vi "State Logic.vi"(0 "TLB' data in":refnum<class "{TMPL} TLB`.lvclass">, 1 "process state logic enable":bool, 5 "trigger queue in":refnum<queue>, 7 "action queue in":refnum<queue>, 11 "error in":errorcluster) -> (4 "TLB' data out":refnum<class "{TMPL} TLB`.lvclass">, 15 "error out":errorcluster)   [LabVIEW 2018, in "TLB` Template.lvlib" / "{TMPL} TLB`.lvclass"]
doc: "Control process for TLB' template.\n\n<B>Input Parameters</B>\n\n<B>TLB' data in</B> is the templates' private data.\n\n<B>process state logic enable</B> enable state logic change.\n\n<B>trigger queue in</B> is a reference to a queue. Use the Create Trigger Queue function to obtain a queue reference. \n\n<B>action queue in</B> is a reference to a queue. Use the Create Action Queue function to obtain a queue reference. \n\n<B>timeout (ms)</B> queue timeout.\n\n<B>error in</B> describes error conditions that occur before this node runs. This input provides standard error in functionality.\n\n<B>Output Parameters</B>\n\n<B>TLB' data out</B> is the templates' private data.\n\n<B>error out</B> contains error information. This output provides standard error out functionality."
uses:
  {TMPL} TLB`.lvclass
  Application Components/Trigger API/System Trigger Element.ctl
  Application Components/Trigger API/System Trigger.ctl
  Core Components/Actions/System Action Element.ctl
  {TMPL} TLB`.lvclass/{TMPL} TLB`.ctl
  State.ctl
  Core Components/Error Handler/TLB` Error Handler.lvclass/TLB` Error Handler.ctl
  Core Components/Error Handler/accessors/Get Action Causing Error.vi
  Core Components/Error Handler/accessors/Get Originating State.vi
  Core Components/Error Handler/accessors/Get Destination State.vi
  Core Components/Error Handler/accessors/Get Executed System Actions.vi
  Core Components/Error Handler/accessors/Get Remaing System Actions.vi
  Core Components/Error Handler/Core/actions/support/Error FLUSH-LOG-DIALOG.vi
  Core Components/Error Handler/Core/actions/support/Error FLUSH-DIALOG.vi
  Application Components/Trigger API/{TMPL} Trigger API.lvlib
  Core Components/Error Handler/TLB` Error Handler.lvclass
  Core Components/Actions/Actions.lvlib
  TLB` Template.lvlib
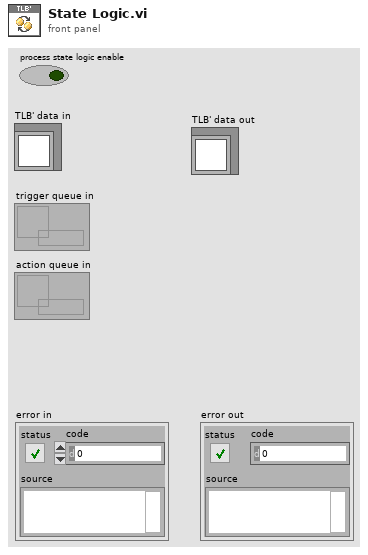
[diagram p1: front panel]
types:
  T1 = typedef "TLB` Template.lvlib/{TMPL} TLB`.lvclass/State.ctl" = enum16{"<Startup>", "Idle", "Connected", "Monitoring", "Sweeping", "<Shutdown>", "<Error>"}
  T2 = typedef "TLB` Template.lvlib/{TMPL} Trigger API.lvlib/System Trigger.ctl" = enum16{"<None>", "Connect", "Start Acquisition", "Stop Acquisition", "Disconnect", "Load Configuration", "Save Configuration", "<Return to Safe State Actions>", "<Cache User Parameters>", "<Close Application>", "<Error>"}
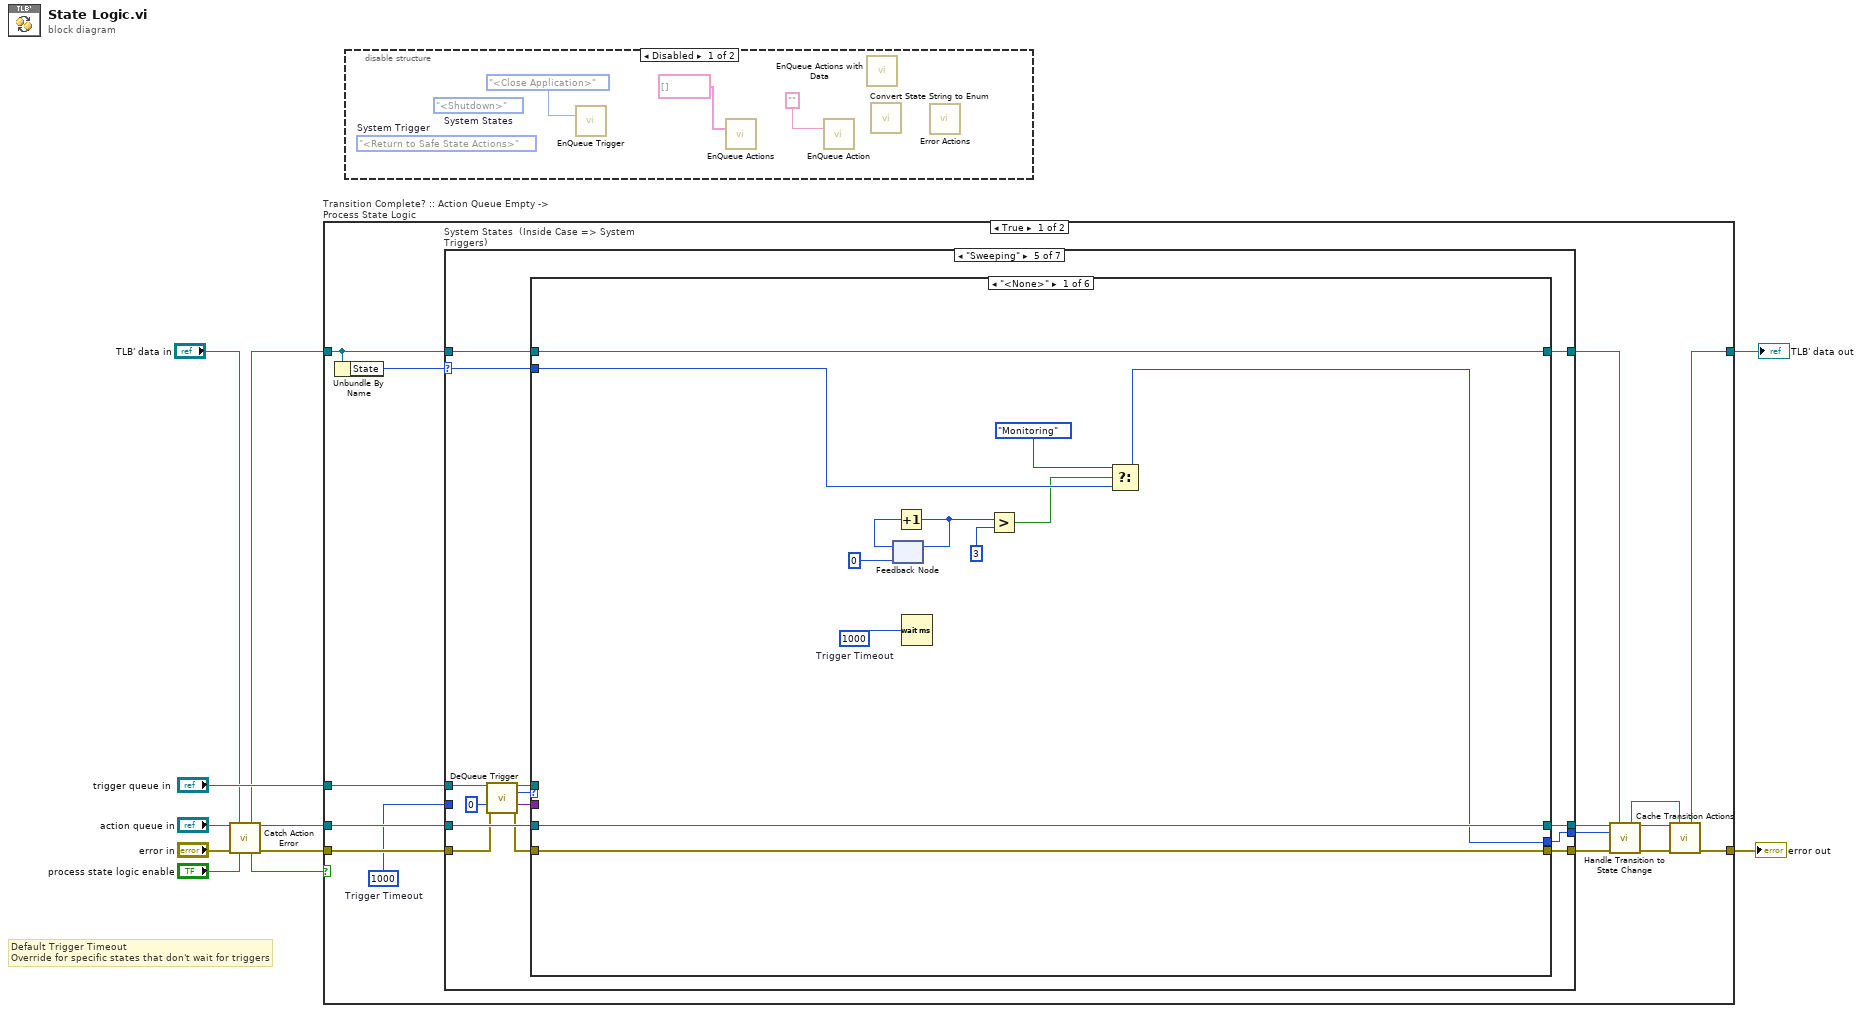
[diagram p0: block diagram]
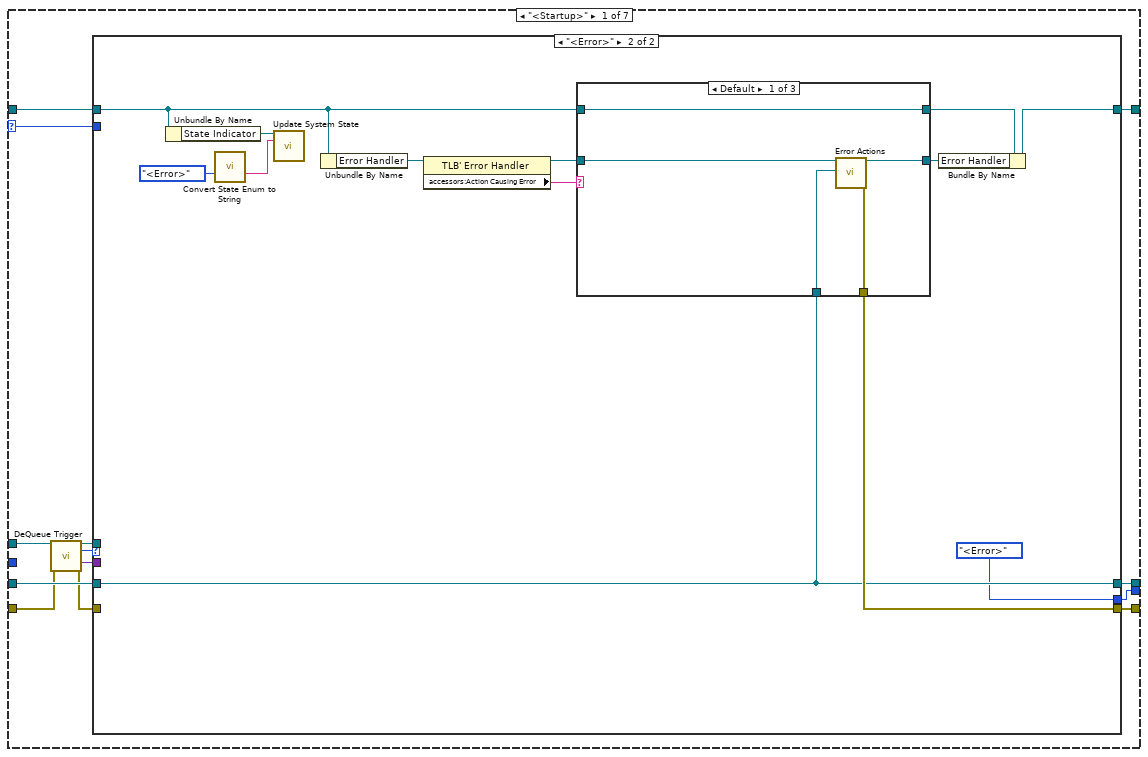
[diagram p3: hidden frame]
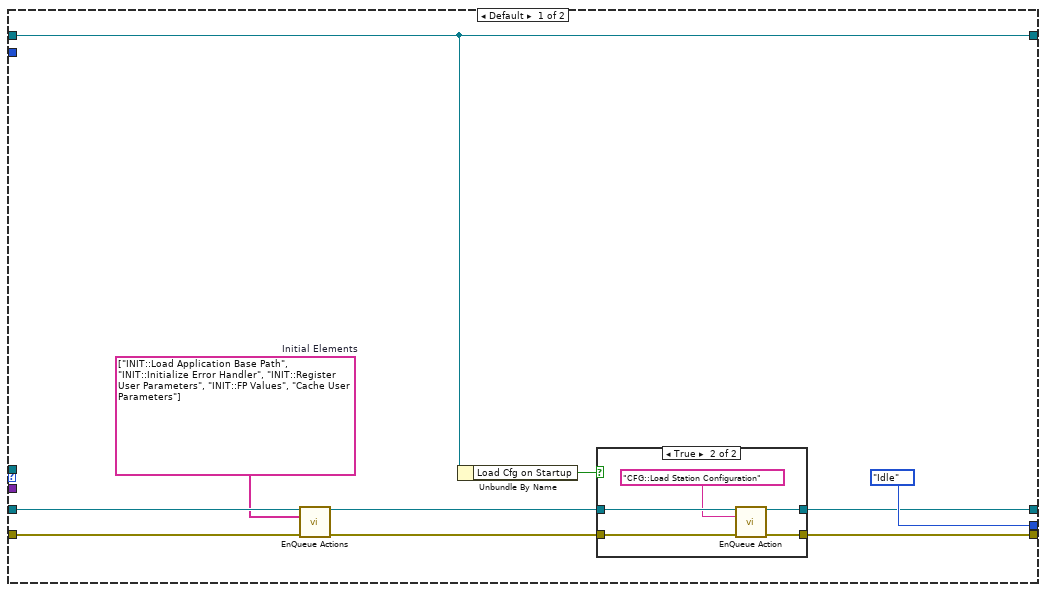
[diagram p4: hidden frame]
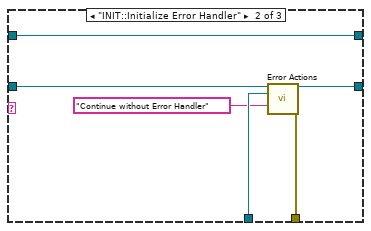
[diagram p6: hidden frame]
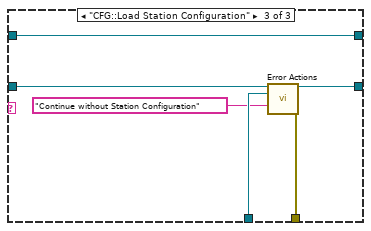
[diagram p7: hidden frame]
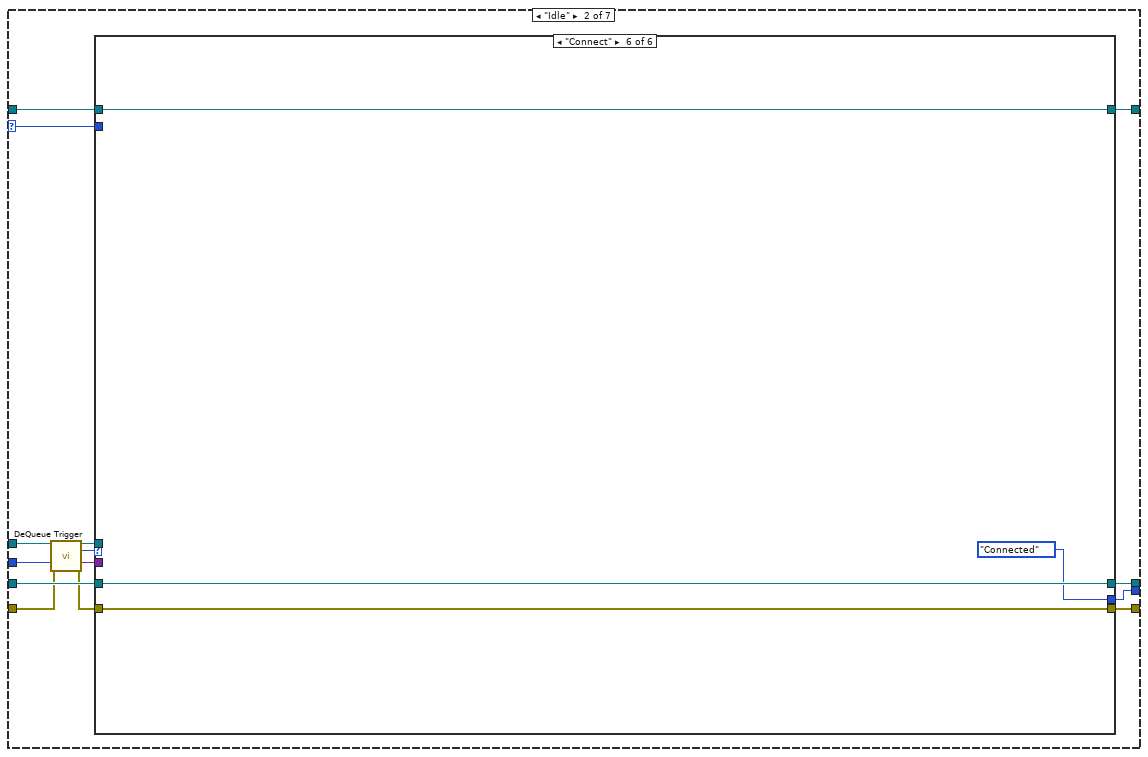
[diagram p8: hidden frame]
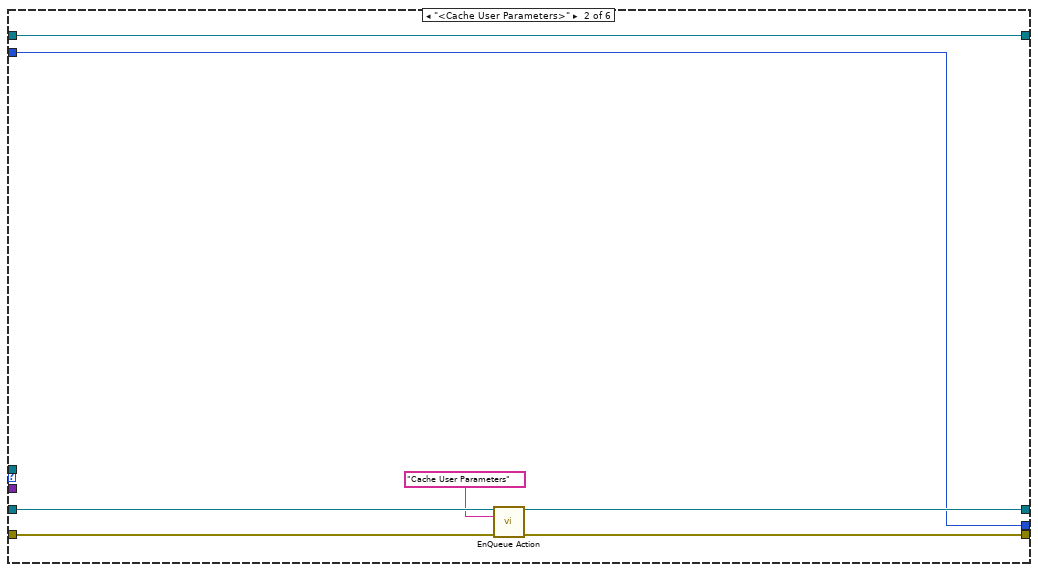
[diagram p10: hidden frame]
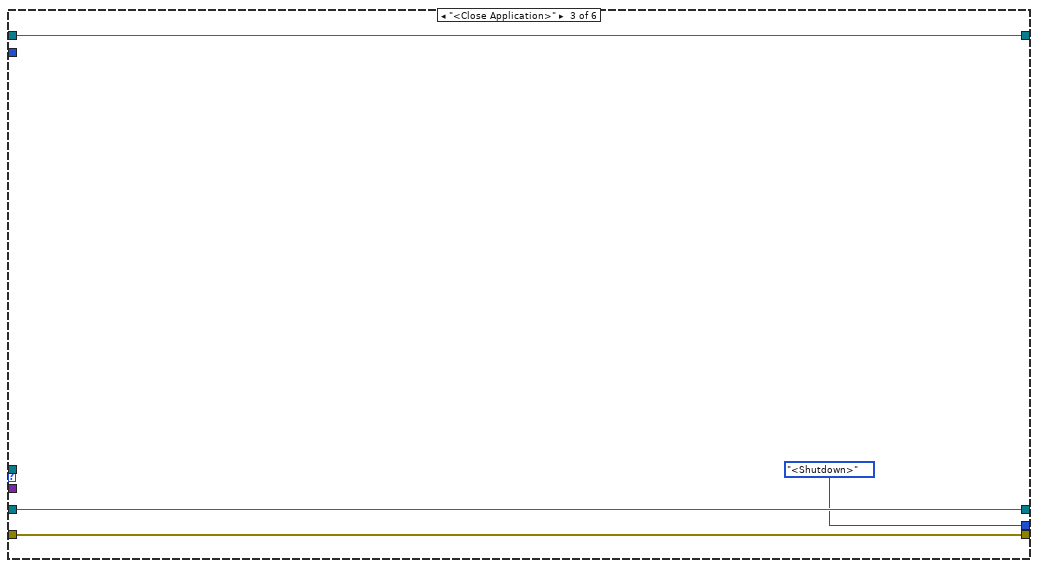
[diagram p11: hidden frame]
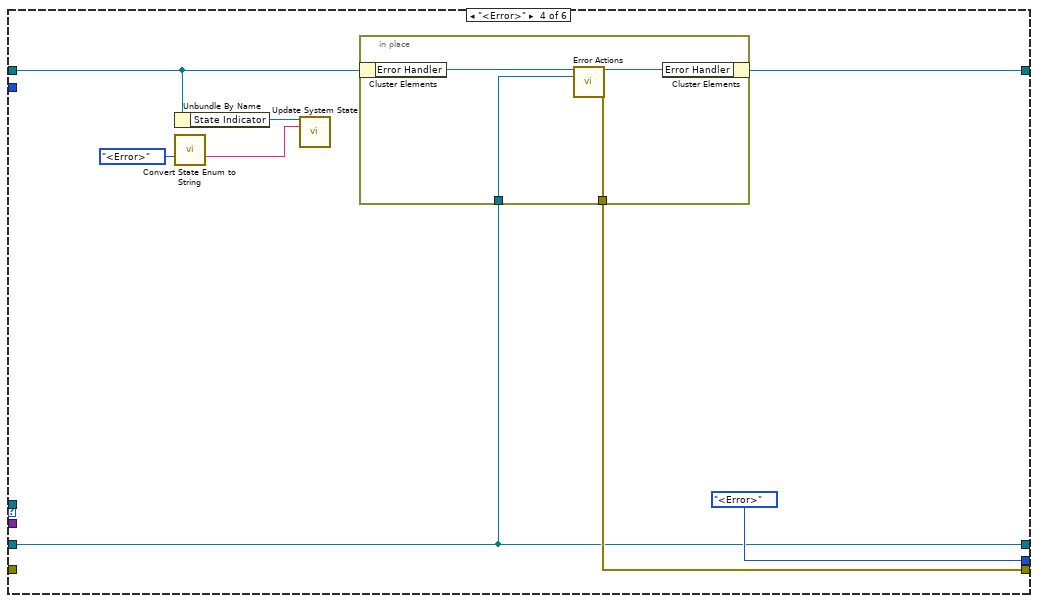
[diagram p12: hidden frame]
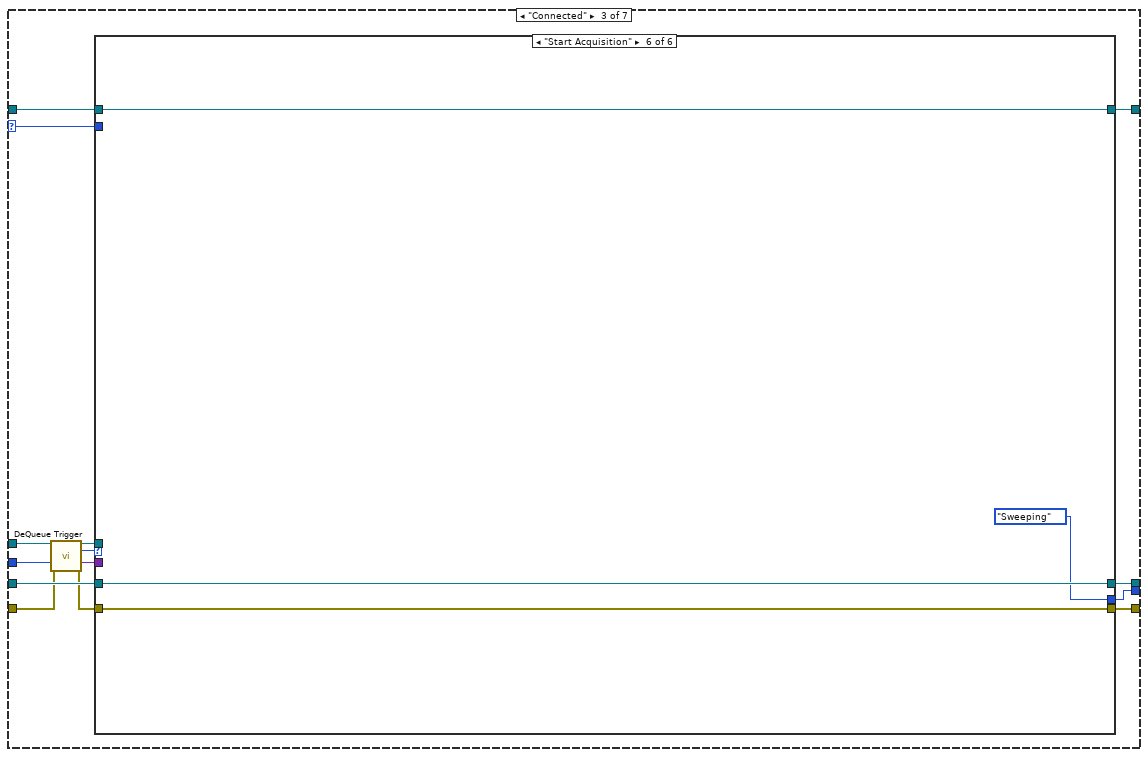
[diagram p14: hidden frame]
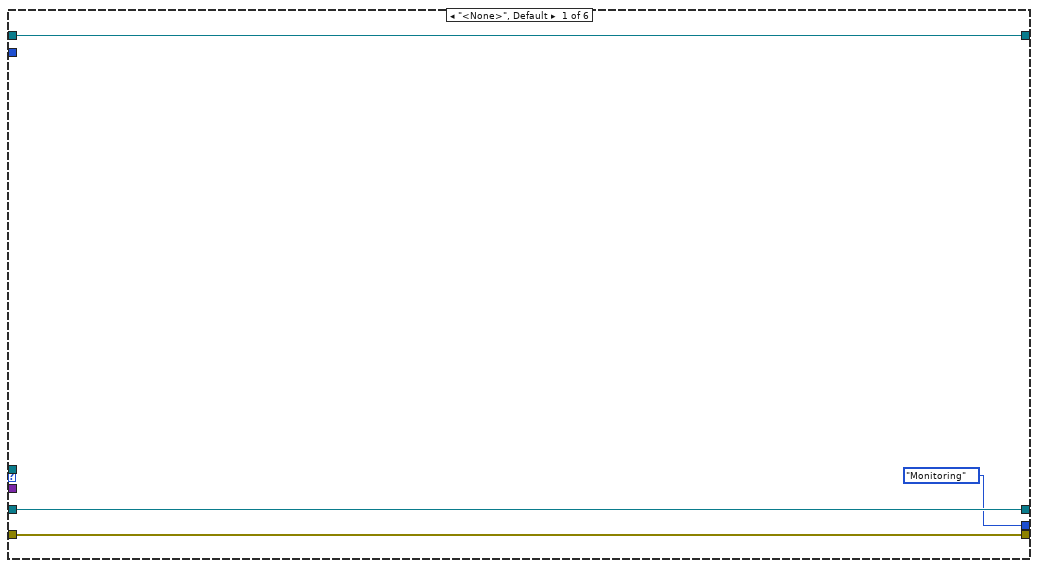
[diagram p15: hidden frame]
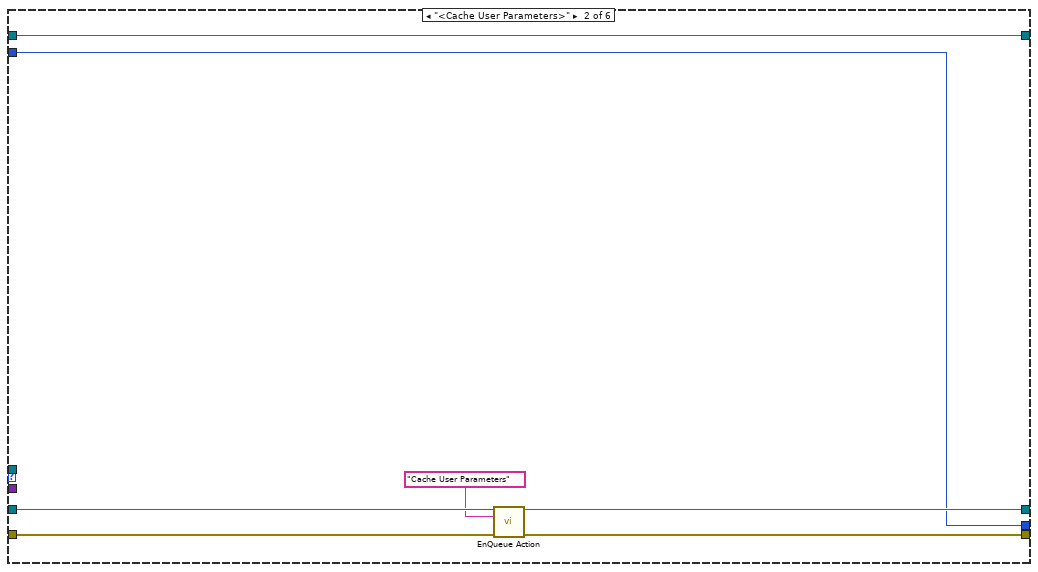
[diagram p16: hidden frame]
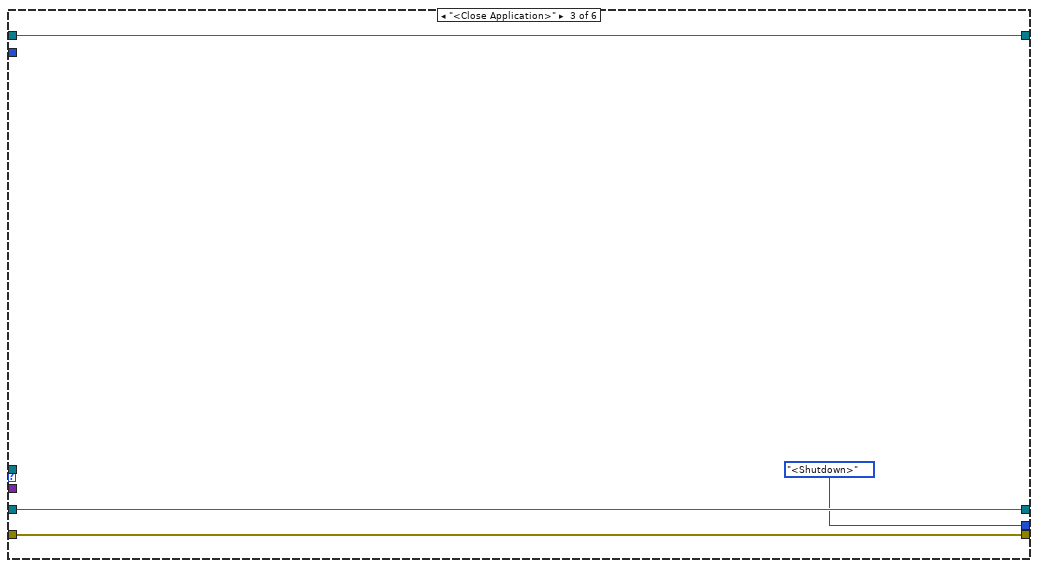
[diagram p17: hidden frame]
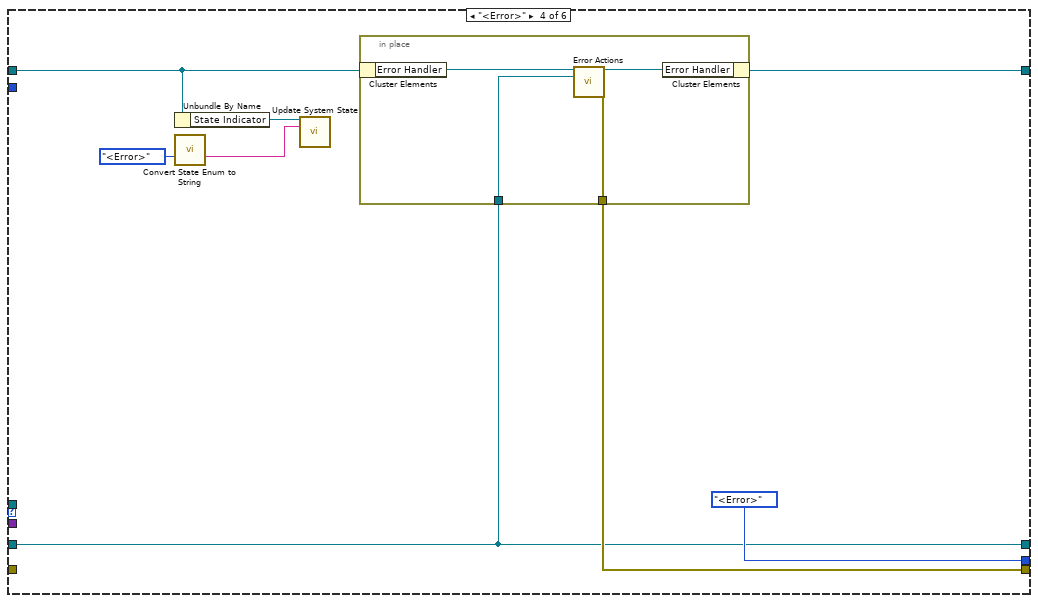
[diagram p18: hidden frame]
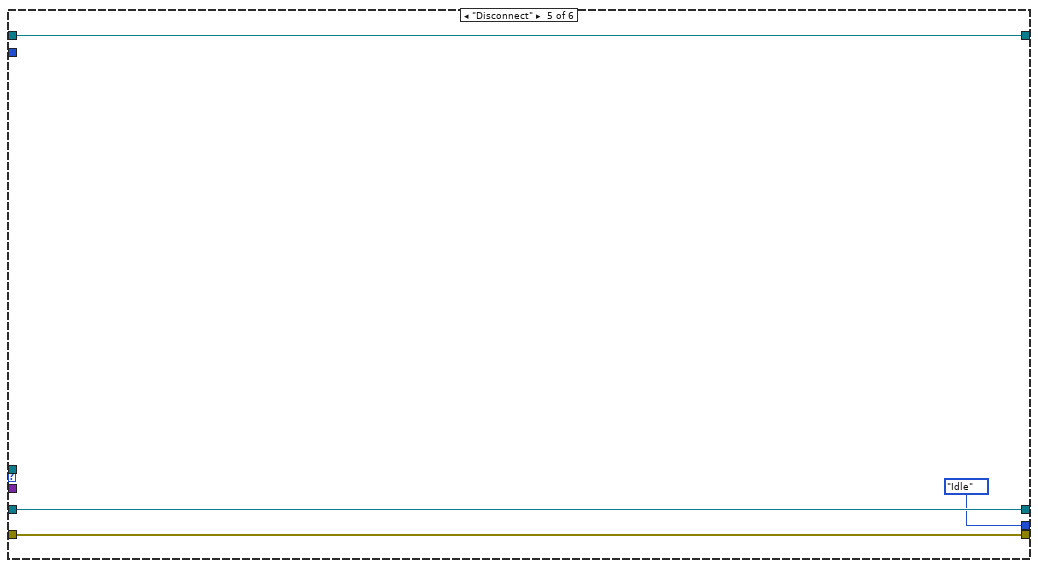
[diagram p19: hidden frame]
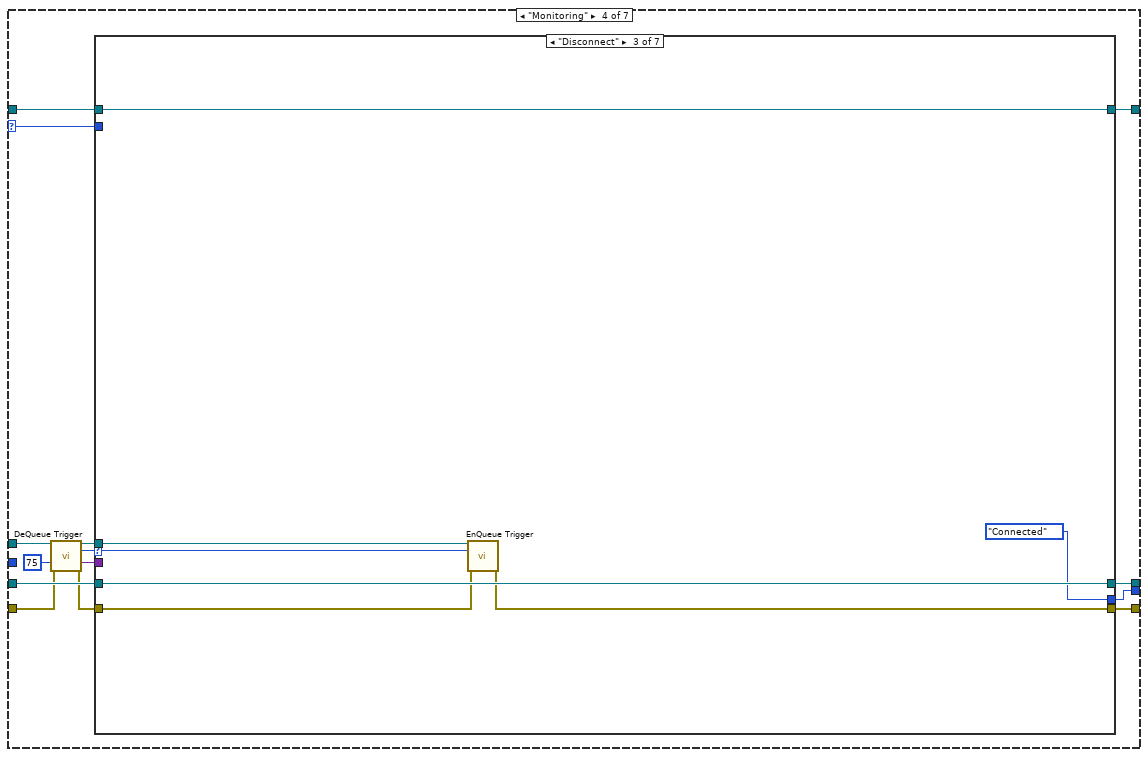
[diagram p20: hidden frame]
diagram:
  # "Default Trigger Timeout\nOverride for specific states that don't wait for triggers"
  n1 = call "Catch Action Error.vi"("action queue in"="action queue in", "TLB' Template in"="TLB' data in", "error in (no error)"="error in", "process state logic enable in"="process state logic enable") -> ("TLB' Template out"=w6:refnum<class "{TMPL} TLB`.lvclass">, "action queue in"=w2:refnum<queue>, "process state logic enable out"=w4:bool, "error out"=w7:errorcluster)  [unwired: 8 in]
  n2 = case "Transition Complete? :: Action Queue Empty -> Process State Logic" shown="True" w4 {
    tunnel: [w17 w404] -> w10
    tunnel: w6 -> [w22 w404]
    tunnel: w7 -> [w26 w405]
    tunnel: w2 -> [w25 _]
    tunnel: [w20 w405] -> w11
    tunnel: "trigger queue in" -> [w24 _]
    frame True {
      w18 = 1000  # Trigger Timeout
      n3 = Unbundle By Name(w22) -> ("State"=w19:T1)
      n4 = case "System States  (Inside Case => System Triggers)" shown="\"Sweeping\"" w19 {
        selector: w19 -> [w27 w89 w138 w187 w243 w305 _]
        tunnel: [w33 w94 w143 w192 w248 w303 w402] -> w15
        tunnel: w22 -> [w34 w95 w144 w193 w249 w304 w402]
        tunnel: w26 -> [w32 w93 w142 w191 w247 w302 w401]
        tunnel: w25 -> [w38 w99 w148 w197 w253 w306 w400]
        tunnel: [w37 w98 w147 w196 w252 w309 w398] -> w23
        tunnel: w24 -> [w39 w100 w149 w198 w254 w310 _]
        tunnel: [w36 w97 w146 w195 w251 w308 w399] -> w16
        tunnel: [w35 w96 w145 w194 w250 w307 State."<Shutdown>" ("State")] -> w12
        tunnel: w18 -> [_ w88 w137 _ _ _ _]
        frame "<Startup>" {
          n5 = call "DeQueue Trigger.vi"("trigger queue in"=w39, "error in"=w32) -> ("trigger queue out"=w28:refnum<queue>, "system trigger"=w30:T2, "trigger data"=w29:variant, "error out"=w31:errorcluster)  [unwired: 10 in]
          n6 = case shown="\"<Error>\"" w30 {
            tunnel: w31 -> [w46 _]
            tunnel: w38 -> [w48 w67]
            tunnel: [w43 w68] -> w37
            tunnel: [w41 w67] -> w36
            tunnel: w29 -> [_ _]
            tunnel: [State."Idle" ("State") State."<Error>" ("State")] -> w35
            tunnel: w34 -> [w44 w58]
            tunnel: [w44 w69] -> w33
            tunnel: w28 -> [_ _]
            tunnel: w27 -> [_ _]
            frame Default {
              w47 = string[] ["INIT::Load Application Base Path", "INIT::Initialize Error Handler", "INIT::Register User Parameters", "INIT::FP Values", "Cache User Parameters"]  # Initial Elements
              n7 = call "EnQueue Actions.vi"("action queue in"=w48, "actions"=w47, "error in"=w46) -> ("action queue out"=w42:refnum<queue>, "error out"=w45:errorcluster)  [unwired: 11 in]
              n8 = Unbundle By Name(w44) -> ("Load Cfg on Startup"=w40:bool)
              n9 = case shown="True" w40 {
                tunnel: w45 -> [w50 w56]
                tunnel: [w50 w55] -> w43
                tunnel: w42 -> [w51 w54]
                tunnel: [w51 w53] -> w41
                frame False {
                }
                frame True {
                  n10 = call "EnQueue Action.vi"("action queue in"=w54, "action"="CFG::Load Station Configuration", "error in"=w56) -> ("action queue out"=w53:refnum<queue>, "error out"=w55:errorcluster)  [unwired: 11 in]
                }
              }
            }
            frame "<Error>" {
              n11 = Unbundle By Name(w58) -> ("State Indicator"=w62:refnum<user-event>)
              n12 = call "Convert State Enum to String.vi"("state in"=State."<Error>") -> ("state out"=w61:string)  [unwired: 13 in, 1 out]
              n13 = call "Update System State.vi"("State Indicator"=w62, "system state message"=w61) -> ()  [unwired: 13 in, 1 out]
              n14 = Unbundle By Name(w58) -> ("Error Handler"=w64:refnum<class "TLB` Error Handler.lvclass">)
              n15 = property class="TLB' Error Handler"(reference=w64) -> (reference out=w63:refnum<class "TLB` Error Handler.lvclass">, "accessors:Action Causing Error"=w60:string)  [unwired: 1 in, 1 out]
              n16 = case shown="Default" w60 {
                tunnel: [w72 w80 w86] -> w68
                tunnel: w67 -> [w71 w79 w85]
                tunnel: [w73 w78 w84] -> w65
                tunnel: w63 -> [w74 w77 w83]
                tunnel: w58 -> [w70 w75 w81]
                tunnel: [w70 w75 w81] -> w57
                frame Default {
                  n17 = call-poly "Error Actions.vi"("Error Handler in"=w74, "action queue in"=w71) -> ("Error Handler out"=w73:refnum<class "TLB` Error Handler.lvclass">, "error out"=w72:errorcluster)  [unwired: 12 in]
                }
                frame "INIT::Initialize Error Handler" {
                  n18 = call-poly "Error Actions.vi"("Error Handler in"=w77, "action queue in"=w79, "error button text (Return to Safe State)"="Continue without Error Handler") -> ("Error Handler out"=w78:refnum<class "TLB` Error Handler.lvclass">, "error out"=w80:errorcluster)  [unwired: 11 in]
                }
                frame "CFG::Load Station Configuration" {
                  n19 = call-poly "Error Actions.vi"("Error Handler in"=w83, "action queue in"=w85, "error button text (Return to Safe State)"="Continue without Station Configuration") -> ("Error Handler out"=w84:refnum<class "TLB` Error Handler.lvclass">, "error out"=w86:errorcluster)  [unwired: 11 in]
                }
              }
              n20 = Bundle By Name(cluster=w57, "Error Handler"=w65) -> (w69:refnum<class "{TMPL} TLB`.lvclass">)
            }
          }
        }
        frame "Idle" {
          n21 = call "DeQueue Trigger.vi"("trigger queue in"=w100, "timeout, ms (0)"=w88, "error in"=w93) -> ("trigger queue out"=w87:refnum<queue>, "system trigger"=w91:T2, "trigger data"=w90:variant, "error out"=w92:errorcluster)  [unwired: 9 in]
          n22 = case shown="\"Connect\"" w91 {
            tunnel: w92 -> [w103 w111 w114 _ w130 w135]
            tunnel: w99 -> [w104 w108 w115 w119 w131 w134]
            tunnel: [w103 w109 w114 w121 w130 w135] -> w98
            tunnel: [w104 w107 w115 w119 w131 w134] -> w97
            tunnel: w90 -> [_ _ _ _ _ _]
            tunnel: w95 -> [w102 w110 w113 w118 w129 w133]
            tunnel: [w101 w105 State."<Shutdown>" ("State") State."<Error>" ("State") w128 State."Connected" ("State")] -> w96
            tunnel: [w102 w110 w113 w120 w129 w133] -> w94
            tunnel: w89 -> [w101 w105 _ _ w128 _]
            tunnel: w87 -> [_ _ _ _ _ _]
            frame "<None>" {
            }
            frame "<Cache User Parameters>" {
              n23 = call "EnQueue Action.vi"("action queue in"=w108, "action"="Cache User Parameters", "error in"=w111) -> ("action queue out"=w107:refnum<queue>, "error out"=w109:errorcluster)  [unwired: 11 in]
            }
            frame "<Close Application>" {
            }
            frame "<Error>" {
              n24 = Unbundle By Name(w118) -> ("State Indicator"=w122:refnum<user-event>)
              n25 = call "Convert State Enum to String.vi"("state in"=State."<Error>") -> ("state out"=w116:string)  [unwired: 13 in, 1 out]
              n26 = call "Update System State.vi"("State Indicator"=w122, "system state message"=w116) -> ()  [unwired: 13 in, 1 out]
              n27 = in-place {
                in-place-border: [w125] -> w121
                in-place-border: w119 -> [w124]
                n28 = in-place-cluster #1(w118) -> ("Error Handler"=w127:refnum<class "TLB` Error Handler.lvclass">)
                n29 = call-poly "Error Actions.vi"("Error Handler in"=w127, "action queue in"=w124) -> ("Error Handler out"=w126:refnum<class "TLB` Error Handler.lvclass">, "error out"=w125:errorcluster)  [unwired: 12 in]
                n30 = in-place-cluster #1("Error Handler"=w126) -> (w120:refnum<class "{TMPL} TLB`.lvclass">)
              }
            }
            frame Default {
            }
            frame "Connect" {
            }
          }
        }
        frame "Connected" {
          n31 = call "DeQueue Trigger.vi"("trigger queue in"=w149, "timeout, ms (0)"=w137, "error in"=w142) -> ("trigger queue out"=w136:refnum<queue>, "system trigger"=w140:T2, "trigger data"=w139:variant, "error out"=w141:errorcluster)  [unwired: 9 in]
          n32 = case shown="\"Start Acquisition\"" w140 {
            tunnel: w141 -> [w152 w160 w163 _ w180 w184]
            tunnel: w148 -> [w153 w157 w164 w168 w179 w183]
            tunnel: [w152 w158 w163 w170 w180 w184] -> w147
            tunnel: [w153 w156 w164 w168 w179 w183] -> w146
            tunnel: w139 -> [_ _ _ _ _ _]
            tunnel: w144 -> [w151 w159 w162 w167 w178 w182]
            tunnel: [State."Monitoring" ("State") w154 State."<Shutdown>" ("State") State."<Error>" ("State") State."Idle" ("State") State."Sweeping" ("State")] -> w145
            tunnel: [w151 w159 w162 w169 w178 w182] -> w143
            tunnel: w138 -> [_ w154 _ _ _ _]
            tunnel: w136 -> [_ _ _ _ _ _]
            frame "<None>", Default {
            }
            frame "<Cache User Parameters>" {
              n33 = call "EnQueue Action.vi"("action queue in"=w157, "action"="Cache User Parameters", "error in"=w160) -> ("action queue out"=w156:refnum<queue>, "error out"=w158:errorcluster)  [unwired: 11 in]
            }
            frame "<Close Application>" {
            }
            frame "<Error>" {
              n34 = Unbundle By Name(w167) -> ("State Indicator"=w171:refnum<user-event>)
              n35 = call "Convert State Enum to String.vi"("state in"=State."<Error>") -> ("state out"=w165:string)  [unwired: 13 in, 1 out]
              n36 = call "Update System State.vi"("State Indicator"=w171, "system state message"=w165) -> ()  [unwired: 13 in, 1 out]
              n37 = in-place {
                in-place-border: [w174] -> w170
                in-place-border: w168 -> [w173]
                n38 = in-place-cluster #2(w167) -> ("Error Handler"=w176:refnum<class "TLB` Error Handler.lvclass">)
                n39 = call-poly "Error Actions.vi"("Error Handler in"=w176, "action queue in"=w173) -> ("Error Handler out"=w175:refnum<class "TLB` Error Handler.lvclass">, "error out"=w174:errorcluster)  [unwired: 12 in]
                n40 = in-place-cluster #2("Error Handler"=w175) -> (w169:refnum<class "{TMPL} TLB`.lvclass">)
              }
            }
            frame "Disconnect" {
            }
            frame "Start Acquisition" {
            }
          }
        }
        frame "Monitoring" {
          n41 = call "DeQueue Trigger.vi"("trigger queue in"=w198, "timeout, ms (0)"=75, "error in"=w191) -> ("trigger queue out"=w186:refnum<queue>, "system trigger"=w189:T2, "trigger data"=w188:variant, "error out"=w190:errorcluster)  [unwired: 9 in]
          n42 = case shown="\"Disconnect\"" w189 {
            selector: w189 -> [_ _ w211 _ _ _ _]
            tunnel: w190 -> [w201 w206 w208 w220 w223 _ w239]
            tunnel: w197 -> [w202 w205 w213 w217 w224 w228 w240]
            tunnel: [w201 w206 w209 w218 w223 w230 w239] -> w196
            tunnel: [w202 w205 w213 w216 w224 w228 w240] -> w195
            tunnel: w188 -> [_ _ _ _ _ _ _]
            tunnel: w193 -> [w200 w204 w212 w219 w222 w227 w238]
            tunnel: [w199 State."Sweeping" ("State") State."Connected" ("State") w214 State."<Shutdown>" ("State") State."<Error>" ("State") w237] -> w194
            tunnel: [w200 w204 w212 w219 w222 w229 w238] -> w192
            tunnel: w187 -> [w199 _ _ w214 _ _ w237]
            tunnel: w186 -> [_ _ w207 _ _ _ _]
            frame "<None>" {
            }
            frame "Start Acquisition" {
            }
            frame "Disconnect" {
              n43 = call "EnQueue Trigger.vi"("trigger queue in"=w207, "system trigger"=w211, "error in"=w208) -> ("error out"=w209:errorcluster)  [unwired: 11 in, 1 out]
            }
            frame "<Cache User Parameters>" {
              n44 = call "EnQueue Action.vi"("action queue in"=w217, "action"="Cache User Parameters", "error in"=w220) -> ("action queue out"=w216:refnum<queue>, "error out"=w218:errorcluster)  [unwired: 11 in]
            }
            frame "<Close Application>" {
            }
            frame "<Error>" {
              n45 = Unbundle By Name(w227) -> ("State Indicator"=w231:refnum<user-event>)
              n46 = call "Convert State Enum to String.vi"("state in"=State."<Error>") -> ("state out"=w225:string)  [unwired: 13 in, 1 out]
              n47 = call "Update System State.vi"("State Indicator"=w231, "system state message"=w225) -> ()  [unwired: 13 in, 1 out]
              n48 = in-place {
                in-place-border: [w234] -> w230
                in-place-border: w228 -> [w233]
                n49 = in-place-cluster #3(w227) -> ("Error Handler"=w236:refnum<class "TLB` Error Handler.lvclass">)
                n50 = call-poly "Error Actions.vi"("Error Handler in"=w236, "action queue in"=w233) -> ("Error Handler out"=w235:refnum<class "TLB` Error Handler.lvclass">, "error out"=w234:errorcluster)  [unwired: 12 in]
                n51 = in-place-cluster #3("Error Handler"=w235) -> (w229:refnum<class "{TMPL} TLB`.lvclass">)
              }
            }
            frame Default {
            }
          }
        }
        frame "Sweeping" {
          n52 = call "DeQueue Trigger.vi"("trigger queue in"=w254, "timeout, ms (0)"=0, "error in"=w247) -> ("trigger queue out"=w242:refnum<queue>, "system trigger"=w245:T2, "trigger data"=w244:variant, "error out"=w246:errorcluster)  [unwired: 9 in]
          n53 = case shown="\"<None>\"" w245 {
            tunnel: w246 -> [w265 w270 w277 w280 _ w296]
            tunnel: w253 -> [w266 w269 w274 w281 w285 w297]
            tunnel: [w265 w270 w275 w280 w287 w296] -> w252
            tunnel: [w266 w269 w273 w281 w285 w297] -> w251
            tunnel: w244 -> [_ _ _ _ _ _]
            tunnel: w249 -> [w264 w268 w276 w279 w284 w295]
            tunnel: [w262 State."Monitoring" ("State") w271 State."<Shutdown>" ("State") State."<Error>" ("State") w294] -> w250
            tunnel: [w264 w268 w276 w279 w286 w295] -> w248
            tunnel: w243 -> [w263 _ w271 _ _ w294]
            tunnel: w242 -> [_ _ _ _ _ _]
            frame "<None>" {
              w255 = 1000  # Trigger Timeout
              n54 = feedback #4(0 ("timeout, ms (0)")) -> (w260:i32)
              n55 = Increment(x=w260) -> (x+1=w258:i32)
              n56 = feedback-in #4(w258) -> ()
              n57 = Wait (ms)(milliseconds to wait=w255) -> ()  [unwired: 1 out]
              n58 = Greater?(x=w258, y=3 ("timeout, ms (0)")) -> (0:w256:bool)
              n59 = Select(t=State."Monitoring", s=w256, f=w263) -> (s? t:f=w262:T1)
            }
            frame "Stop Acquisition" {
            }
            frame "<Cache User Parameters>" {
              n60 = call "EnQueue Action.vi"("action queue in"=w274, "action"="Cache User Parameters", "error in"=w277) -> ("action queue out"=w273:refnum<queue>, "error out"=w275:errorcluster)  [unwired: 11 in]
            }
            frame "<Close Application>" {
            }
            frame "<Error>" {
              n61 = Unbundle By Name(w284) -> ("State Indicator"=w288:refnum<user-event>)
              n62 = call "Convert State Enum to String.vi"("state in"=State."<Error>") -> ("state out"=w282:string)  [unwired: 13 in, 1 out]
              n63 = call "Update System State.vi"("State Indicator"=w288, "system state message"=w282) -> ()  [unwired: 13 in, 1 out]
              n64 = in-place {
                in-place-border: [w291] -> w287
                in-place-border: w285 -> [w290]
                n65 = in-place-cluster #5(w284) -> ("Error Handler"=w293:refnum<class "TLB` Error Handler.lvclass">)
                n66 = call-poly "Error Actions.vi"("Error Handler in"=w293, "action queue in"=w290) -> ("Error Handler out"=w292:refnum<class "TLB` Error Handler.lvclass">, "error out"=w291:errorcluster)  [unwired: 12 in]
                n67 = in-place-cluster #5("Error Handler"=w292) -> (w286:refnum<class "{TMPL} TLB`.lvclass">)
              }
            }
            frame Default {
            }
          }
        }
        frame "<Error>" {
          n68 = call "DeQueue Trigger.vi"("trigger queue in"=w310, "error in"=w302) -> ("trigger queue out"=w301:refnum<queue>, "system trigger"=w300:T2, "trigger data"=w298:variant, "error out"=w299:errorcluster)  [unwired: 10 in]
          n69 = case shown="\"<Close Application>\"" w300 {
            tunnel: w304 -> [w312 w315 w378 w394]
            tunnel: [w313 w325 w387 w393] -> w309
            tunnel: w299 -> [w313 w327 w388 w393]
            tunnel: w306 -> [w314 w328 w389 w396]
            tunnel: [w314 w326 w384 w396] -> w308
            tunnel: [w311 w324 w386 State."<Shutdown>" ("State")] -> w307
            tunnel: w301 -> [_ _ _ _]
            tunnel: w305 -> [w311 _ _ _]
            tunnel: w298 -> [_ _ _ _]
            tunnel: [w312 w323 w378 w394] -> w303
            frame Default {
            }
            frame "<Return to Safe State Actions>" {
              n70 = Unbundle By Name(w315) -> ("Error Handler"=w322:refnum<class "TLB` Error Handler.lvclass">)
              n71 = property class="TLB' Error Handler"(reference=w322) -> ("accessors:Originating State"=w317:string, "accessors:Action Causing Error"=w321:string, "accessors:Destination State"=w320:string, "accessors:Executed System Actions"=w319:string[], "accessors:Remaing System Actions"=w316:string[])  [unwired: 1 in, 2 out]
              n72 = call "Convert State String to Enum.vi"("state in"=w317) -> ("state out"=w318:T1)  [unwired: 13 in, 1 out]
              n73 = case shown="\"<Startup>\"" w318 {
                selector: w318 -> [w329 w336 _]
                tunnel: w328 -> [w332 w342 w375]
                tunnel: w327 -> [w330 w343 w374]
                tunnel: [w330 w341 w374] -> w325
                tunnel: [w332 w340 w375] -> w326
                tunnel: [w329 w339 State."<Shutdown>" ("State")] -> w324
                tunnel: w315 -> [w331 w333 w377]
                tunnel: [w331 w334 w377] -> w323
                tunnel: w321 -> [_ w338 _]
                tunnel: w320 -> [_ w335 _]
                tunnel: w319 -> [_ _ _]
                tunnel: w316 -> [_ w337 _]
                frame Default {
                }
                frame "<Startup>" {
                  n74 = case shown="\"INIT::Initialize Error Handler\"" w338 {
                    tunnel: w343 -> [w346 w359 w372]
                    tunnel: w342 -> [w347 w360 w373]
                    tunnel: [w346 w358 w371] -> w341
                    tunnel: [w347 w357 w370] -> w340
                    tunnel: [State."<Shutdown>" ("State") State."Idle" ("state out") State."Idle" ("state out")] -> w339
                    tunnel: w337 -> [_ w356 w369]
                    tunnel: w336 -> [_ w348 w362]
                    tunnel: w335 -> [_ _ _]
                    tunnel: w333 -> [w344 w350 w363]
                    tunnel: [w344 w349 w361] -> w334
                    frame Default {
                    }
                    frame "INIT::Initialize Error Handler" {
                      n75 = Search 1D Array(1D array=w356, element="Change State") -> (index of element=w354:i32)  [unwired: 1 in]
                      n76 = Delete From Array(array=w356, length=1, index=w354) -> (array with subset deleted=w355:string[])  [unwired: 1 out]
                      n77 = call "EnQueue Actions.vi"("action queue in"=w360, "actions"=w355, "error in"=w359) -> ("action queue out"=w357:refnum<queue>, "error out"=w358:errorcluster)  [unwired: 11 in]
                      n78 = Bundle By Name(cluster=w350, "State"=w348) -> (w349:refnum<class "{TMPL} TLB`.lvclass">)
                    }
                    frame "CFG::Load Station Configuration" {
                      n79 = Search 1D Array(1D array=w369, element="Change State") -> (index of element=w367:i32)  [unwired: 1 in]
                      n80 = Delete From Array(array=w369, length=1, index=w367) -> (array with subset deleted=w368:string[])  [unwired: 1 out]
                      n81 = call "EnQueue Actions.vi"("action queue in"=w373, "actions"=w368, "error in"=w372) -> ("action queue out"=w370:refnum<queue>, "error out"=w371:errorcluster)  [unwired: 11 in]
                      n82 = Bundle By Name(cluster=w363, "State"=w362) -> (w361:refnum<class "{TMPL} TLB`.lvclass">)
                    }
                  }
                }
                frame "<Shutdown>" {
                }
              }
            }
            frame "<Close Application>" {
              n83 = Unbundle By Name(w378) -> ("Error Handler"=w385:refnum<class "TLB` Error Handler.lvclass">)
              n84 = property class="TLB' Error Handler"(reference=w385) -> ("accessors:Originating State"=w383:string, "accessors:Action Causing Error"=w379:string, "accessors:Destination State"=w380:string, "accessors:Executed System Actions"=w381:string[])  [unwired: 1 in, 2 out]
              n85 = call "Convert State String to Enum.vi"("state in"=w383) -> ("state out"=w382:T1)  [unwired: 13 in, 1 out]
              n86 = case shown="Default" w382 {
                tunnel: w389 -> [w391]
                tunnel: w388 -> [w390]
                tunnel: [w390] -> w387
                tunnel: [w391] -> w384
                tunnel: [State."<Shutdown>" ("State")] -> w386
                tunnel: w379 -> [_]
                tunnel: w380 -> [_]
                tunnel: w381 -> [_]
                frame Default {
                }
              }
            }
            frame "<Error>" {
              # "If error errors' that is probably really bad and we should end the program"
            }
          }
        }
        frame "<Shutdown>" {
          n87 = call "EnQueue Actions.vi"("action queue in"=w400, "actions"=string[] ["Exit"], "error in"=w401) -> ("action queue out"=w399:refnum<queue>, "error out"=w398:errorcluster)  [unwired: 11 in]
        }
      }
      n88 = call "Handle Transition to State Change.vi"("action queue in"=w16, "TLB' Template in"=w15, "Destination State"=w12, "error in (no error)"=w23) -> ("TLB' Template out"=w14:refnum<class "{TMPL} TLB`.lvclass">, "action queue in"=w13:refnum<queue>, "error out"=w21:errorcluster)  [unwired: 9 in]
      n89 = call "Cache Transition Actions.vi"("action queue in"=w13, "TLB' Template in"=w14, "error in (no error)"=w21) -> ("TLB' Template out"=w17:refnum<class "{TMPL} TLB`.lvclass">, "error out"=w20:errorcluster)  [unwired: 11 in]
    }
    frame False {
    }
  }
  "error out" <- w11
  "TLB' data out" <- w10
  n90 = disable-structure shown="Disabled" {
    frame Disabled {
      (unwired) System_Trigger."<Return to Safe State Actions>"  # System Trigger
      (unwired) State."<Shutdown>"  # System States
      n91 = call "EnQueue Trigger.vi"("system trigger"=System_Trigger."<Close Application>" ("System Trigger")) -> ()  [unwired: 13 in, 2 out]
      n92 = call "EnQueue Actions.vi"("actions"=string[] [] ("message names")) -> ()  [unwired: 13 in, 2 out]
      n93 = call "EnQueue Action.vi"("action"="" ("Message Name")) -> ()  [unwired: 13 in, 2 out]
      n94 = call "EnQueue Actions with Data.vi"() -> ()  [unwired: 14 in, 2 out]
      n95 = call "Convert State String to Enum.vi"() -> ()  [unwired: 14 in, 2 out]
      n96 = call-poly "Error Actions.vi"() -> ()  [unwired: 14 in, 2 out]
    }
    frame Enabled {
    }
  }
